vi "FileVersionInfo.vi"(8 "error in (no error)":errorcluster, 11 "Application Path in":path) -> (0 "error out":errorcluster, 1 "FileVersionInfo Out":T1, 2 "File Version Info":string, 3 "Application Path out":path)   [LabVIEW 2018]
doc: "This VI obtains information about an existing executable or DLL (such as its version and product name). It can be called as a subVI from a VI that will be built into an executable to obtain information about that executable.\n\nTo obtain version information about an existing executable or DLL, enter a path to an application into \"Application Path in\" and run the VI."
uses:
  <vilib>/Platform/fileVersionInfo.llb/FileVersionInformation.ctl
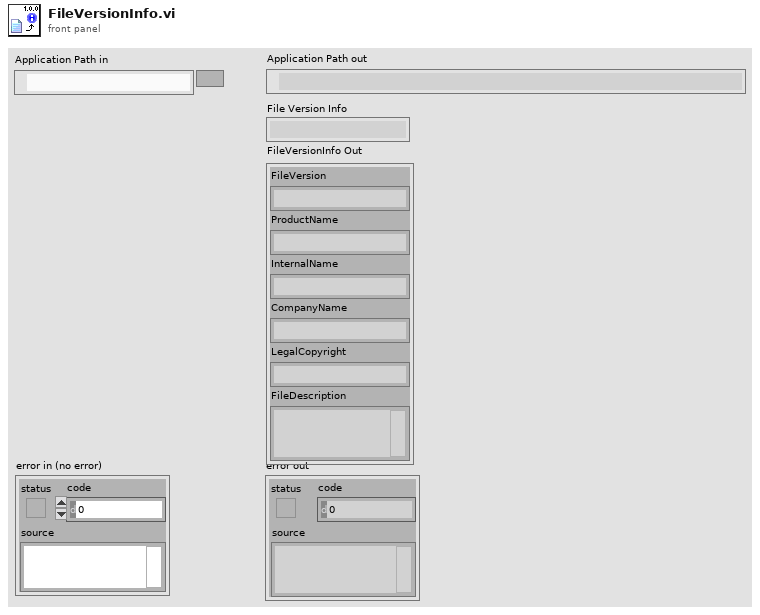
[diagram p1: front panel]
types:
  T1 = typedef "FileVersionInformation.ctl" = cluster{"FileVersion":string, "ProductName":string, "InternalName":string, "CompanyName":string, "LegalCopyright":string, "FileDescription":string}
  T2 = enum16{"CharacterArray", "FixedFileInfoCluster", "LanguageCode"}
  T3 = cluster{"[0]":string, "[1]":string, "[2]":string, "[3]":string, "[4]":string, "[5]":string}
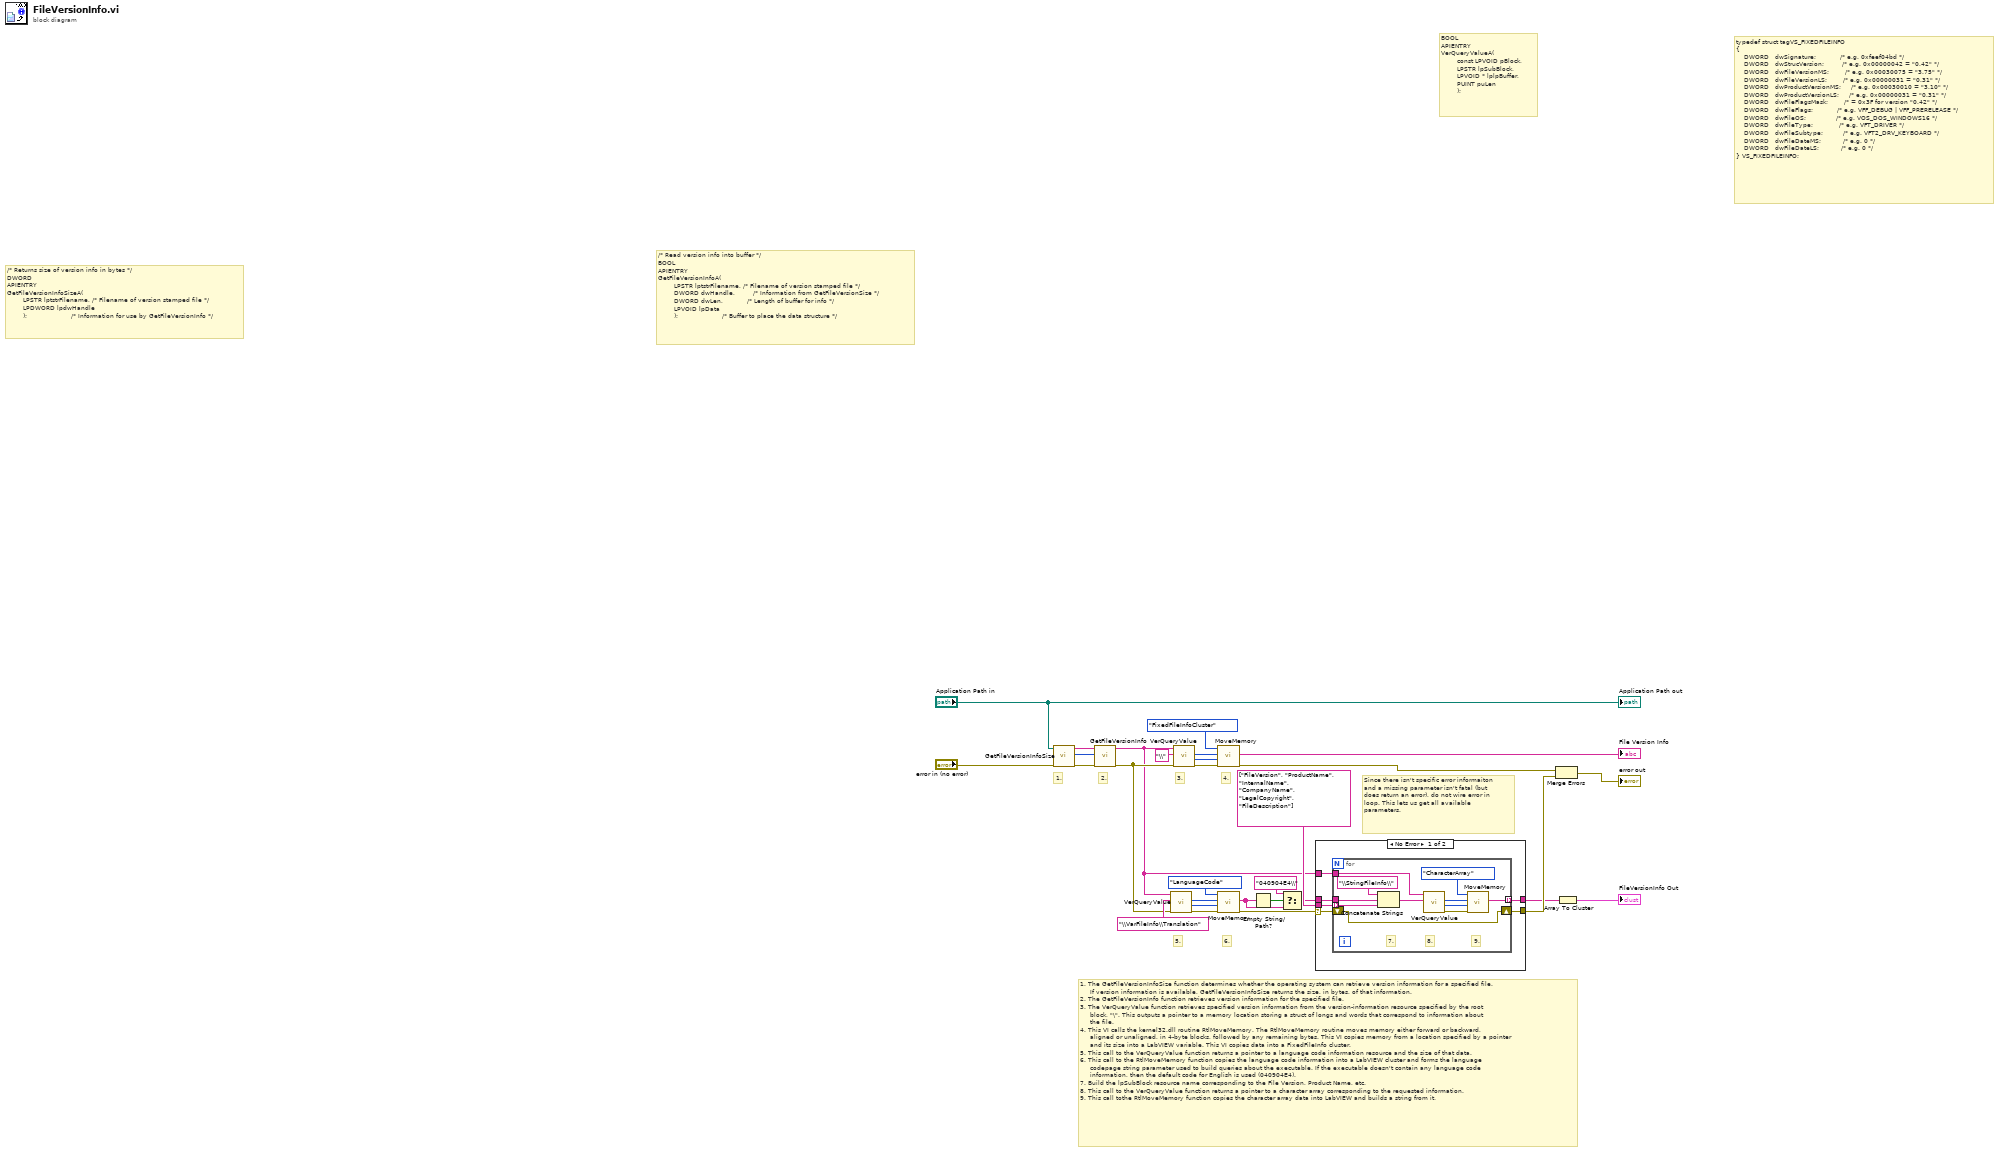
[diagram p0: block diagram]
diagram:
  # "Since there isn't specific error informaiton and a missing parameter isn't fatal (but does return an error), do not wire error in loop. This lets us get all available parameters."
  # "6."
  # "4."
  # "5."
  # "3."
  # "2."
  # "1. The GetFileVersionInfoSize function determines whether the operating system can retrieve version information for a specified file.\n     If version information is available, GetFileVersionInfoSize returns the size, in bytes, of that information.\n2. The GetFileVersionInfo function retrieves version information for the specified file.\n3. The VerQueryValue function retrieves specified version information from the version-information resource specified by the root\n     block, \"\\\". This outputs a pointer to a memory location storing a struct of longs and words that correspond to information about\n     the file.\n4. This VI calls the kernel32.dll routine RtlMoveMemory. The RtlMoveMemory routine moves memory either forward or backward,\n     aligned or unaligned, in 4-byte blocks, followed by any remaining bytes. This VI copies memory from a location specified by a pointer\n     and its size into a LabVIEW variable. This VI copies data into a FixedFileInfo cluster. \n5. This call to the VerQueryValue function returns a pointer to a language code information resource and the size of that data.\n6. This call to the RtlMoveMemory function copies the language code information into a LabVIEW cluster and forms the language\n     codepage string parameter used to build queries about the executable. If the executable doesn't contain any language code\n     information, then the default code for English is used (040904E4).\n7. Build the lpSubBlock resource name corresponding to the File Version, Product Name, etc. \n8. This call to the VerQueryValue function returns a pointer to a character array corresponding to the requested information.\n9. This call tothe RtlMoveMemory function copies the character array data into LabVIEW and builds a string from it."
  # "1."
  # "/* Returns size of version info in bytes */\nDWORD\nAPIENTRY\nGetFileVersionInfoSizeA(\n        LPSTR lptstrFilename, /* Filename of version stamped file */\n        LPDWORD lpdwHandle\n        );                      /* Information for use by GetFileVersionInfo */"
  # "typedef struct tagVS_FIXEDFILEINFO\n{\n    DWORD   dwSignature;            /* e.g. 0xfeef04bd */\n    DWORD   dwStrucVersion;         /* e.g. 0x00000042 = \"0.42\" */\n    DWORD   dwFileVersionMS;        /* e.g. 0x00030075 = \"3.75\" */\n    DWORD   dwFileVersionLS;        /* e.g. 0x00000031 = \"0.31\" */\n    DWORD   dwProductVersionMS;     /* e.g. 0x00030010 = \"3.10\" */\n    DWORD   dwProductVersionLS;     /* e.g. 0x00000031 = \"0.31\" */\n    DWORD   dwFileFlagsMask;        /* = 0x3F for version \"0.42\" */\n    DWORD   dwFileFlags;            /* e.g. VFF_DEBUG | VFF_PRERELEASE */\n    DWORD   dwFileOS;               /* e.g. VOS_DOS_WINDOWS16 */\n    DWORD   dwFileType;             /* e.g. VFT_DRIVER */\n    DWORD   dwFileSubtype;          /* e.g. VFT2_DRV_KEYBOARD */\n    DWORD   dwFileDateMS;           /* e.g. 0 */\n    DWORD   dwFileDateLS;           /* e.g. 0 */\n} VS_FIXEDFILEINFO;"
  # "/* Read version info into buffer */\nBOOL\nAPIENTRY\nGetFileVersionInfoA(\n        LPSTR lptstrFilename, /* Filename of version stamped file */\n        DWORD dwHandle,         /* Information from GetFileVersionSize */\n        DWORD dwLen,            /* Length of buffer for info */\n        LPVOID lpData\n        );                      /* Buffer to place the data structure */"
  # "BOOL\nAPIENTRY\nVerQueryValueA(\n        const LPVOID pBlock,\n        LPSTR lpSubBlock,\n        LPVOID * lplpBuffer,\n        PUINT puLen\n        );"
  n1 = call <vilib>:"GetFileVersionInfoSize.vi"("error in (no error)"="error in (no error)", "Path"="Application Path in") -> ("error out"=w14:errorcluster, "Size"=w13:i32, "lptstrFilename"=w15:string)  [unwired: 7 in]
  n2 = call <vilib>:"GetFileVersionInfo.vi"("error in"=w14, "Size"=w13, "lptstrFilename"=w15) -> ("error out"=w17:errorcluster, "lpData"=w6:string)  [unwired: 7 in]
  n3 = call <vilib>:"VerQueryValue.vi"("error in (no error)"=w17, "lpSubBlock"="\\VarFileInfo\\Translation", "lpData"=w6) -> ("error out"=w18:errorcluster, "puLen"=w20:u32, "lplpBuffer"=w19:u64)  [unwired: 6 in]
  n4 = call <vilib>:"VerQueryValue.vi"("error in (no error)"=w17, "lpSubBlock"="\\", "lpData"=w6) -> ("error out"=w27:errorcluster, "puLen"=w24:u32, "lplpBuffer"=w25:u64)  [unwired: 6 in]
  n5 = call <vilib>:"MoveMemory.vi"("error in (no error)"=w27, "puLen"=w24, "lplpBuffer"=w25, "Datatype"=T2."FixedFileInfoCluster") -> ("error out"=w10:errorcluster, "data"=→"File Version Info":string)  [unwired: 6 in]
  n6 = call <vilib>:"MoveMemory.vi"("error in (no error)"=w18, "puLen"=w20, "lplpBuffer"=w19, "Datatype"=T2."LanguageCode") -> ("error out"=w16:errorcluster, "data"=w4:string)  [unwired: 6 in]
  n7 = Empty String/Path?(string/path=w4) -> (empty?=w5:bool)
  n8 = Select(t="040904E4\\", s=w5, f=w4) -> (s? t:f=w2:string)
  n9 = case shown="No Error" w16 {
    selector: w16 -> [w34 w47]
    tunnel: string[] ["FileVersion", "ProductName", "InternalName", "CompanyName", "LegalCopyright", "FileDescription"] -> [w35 _]
    tunnel: [w33 w47] -> w11
    tunnel: [w32 _] -> w8
    tunnel: w6 -> [w31 _]
    tunnel: w2 -> [w30 _]
    frame No Error {
      n10 = for {
        tunnel: w31 -> [w43]
        tunnel: w35 -> [w45] mode=indexing
        tunnel: [w39] -> w32 mode=indexing
        tunnel: w30 -> [w38]
        shift-right: [w37] -> w33
        shift-left: w34 -> [w37]
        # "7."
        # "9."
        # "8."
        n11 = Concatenate Strings("\\StringFileInfo\\" ("lpSubBlock"), w38, w45) -> (w44:string)
        n12 = call <vilib>:"VerQueryValue.vi"("lpSubBlock"=w44, "lpData"=w43) -> ("error out"=w36:errorcluster, "puLen"=w40:u32, "lplpBuffer"=w41:u64)  [unwired: 7 in]
        n13 = call <vilib>:"MoveMemory.vi"("error in (no error)"=w36, "puLen"=w40, "lplpBuffer"=w41, "Datatype"=T2."CharacterArray") -> ("data"=w39:string)  [unwired: 6 in, 1 out]
      }
    }
    frame Error {
    }
  }
  n14 = Merge Errors(w10, w11) -> (→"error out":errorcluster)
  n15 = Array To Cluster(array=w8) -> (cluster=→"FileVersionInfo Out":T3)
  "Application Path out" <- "Application Path in"
